vi "GLdrv_INFO_CH.vi"(0 "Connection ID":T1, 11 "error in (no error)":errorcluster) -> (4 "Connection ID Out":T1, 6 "Analog Size out":i32, 15 "error out":errorcluster)   [LabVIEW 2017, in "GL860_Driver.lvlib"]
doc: "記録計本体に接続されているアナログCHの数を参照します。"
uses:
  GL860_Driver.lvlib
  ConnectionID.ctl
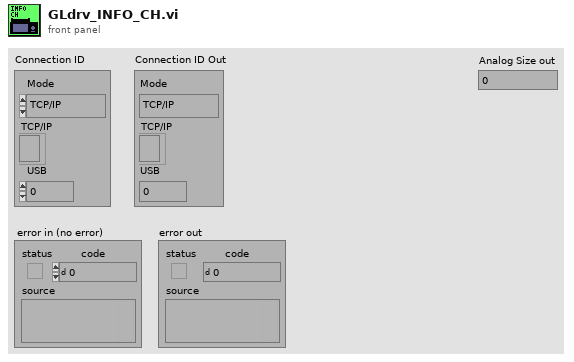
[diagram p1: front panel]
types:
  T1 = typedef "ConnectionID.ctl" = cluster{"Mode":enum16{"TCP/IP", "USB"}, "TCP/IP":refnum<k5>, "USB":i32}
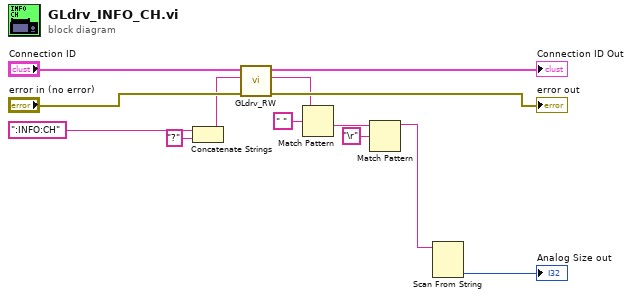
[diagram p0: block diagram]
diagram:
  n1 = Concatenate Strings(":INFO:CH" ("Command"), "?" ("string")) -> (w2:string)
  n2 = call "GLdrv_RW.vi"("error in (no error)"="error in (no error)", "data in"=w2, "Connection ID"="Connection ID") -> ("error out"=→"error out":errorcluster, "data out"=w1:string, "Connection ID Out"=→"Connection ID Out":T1)  [unwired: 4 in, 2 out]
  n3 = Match Pattern(string=w1, regular expression=" " ("search string/char (-)")) -> (after substring=w5:string)  [unwired: 4 out]
  n4 = Match Pattern(string=w5, regular expression="\r") -> (before substring=w3:string)  [unwired: 4 out]
  n5 = Scan From String(input string=w3) -> (output 1=→"Analog Size out":i32)  [unwired: 3 in, 4 out]
